vi "FreqC.Set Threshold.vi"(8 "error In":errorcluster, 10 "Threshold, V":dbl, 11 "FreqC Session in":T1) -> (0 "error out":errorcluster, 3 "FreqC Session out":T1)   [LabVIEW 2018]
uses:
  typedefs/FreqC.Session.ctl
  <instrlib>/Agilent 532XX Series/Public/Configure/Configure Channel (Threshold Voltage).vi
  <instrlib>/Agilent 532XX Series/Agilent 532XX Series.lvlib
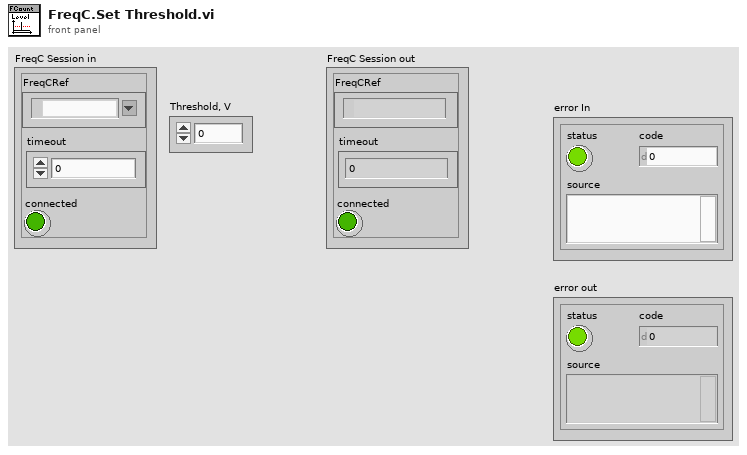
[diagram p1: front panel]
types:
  T1 = typedef "FreqC.Session.ctl" = cluster{"FreqCRef":refnum<visa-resource-name>, "timeout":dbl, "connected":bool}
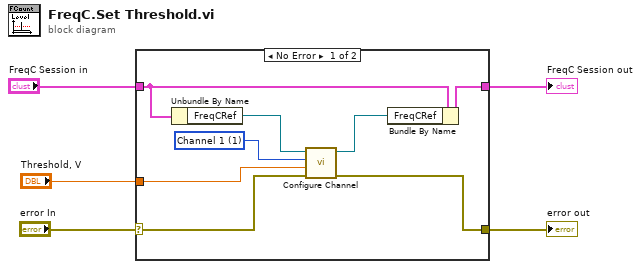
[diagram p0: block diagram]
diagram:
  n1 = case shown="No Error" "error In" {
    selector: "error In" -> [w8 w15]
    tunnel: [w9 w15] -> w4
    tunnel: "FreqC Session in" -> [w13 w14]
    tunnel: "Threshold, V" -> [w6 _]
    tunnel: [w12 w14] -> w1
    frame No Error {
      w7 = 1 items=["Channel 1"=1, "Channel 2"=2] ("Channel (1: Channel 1)")
      n2 = Unbundle By Name(w13) -> ("FreqCRef"=w11:refnum<visa-resource-name>)
      n3 = call-poly <instrlib>:"Configure Channel.vi"("error in (no error)"=w8, "Threshold Voltage (0 V)"=w6, "Channel (1: Channel 1)"=w7, "VISA resource name"=w11) -> ("error out"=w9:errorcluster, "VISA resource name out"=w10:refnum<visa-resource-name>)  [unwired: 6 in]
      n4 = Bundle By Name(cluster=w13, "FreqCRef"=w10) -> (w12:T1)
    }
    frame Error {
    }
  }
  "error out" <- w4
  "FreqC Session out" <- w1
